vi "TDMS_LogMeasurements.vi"(8 "error in (no error)":errorcluster, 9 "Current Time":timestamp, 10 "Motor Measurements":T1, 11 "tdms file":refnum<k34>) -> (0 "error out":errorcluster, 3 "tdms file out":refnum<k34>)   [LabVIEW 2026]
uses:
  MotorMeasurements.ctl
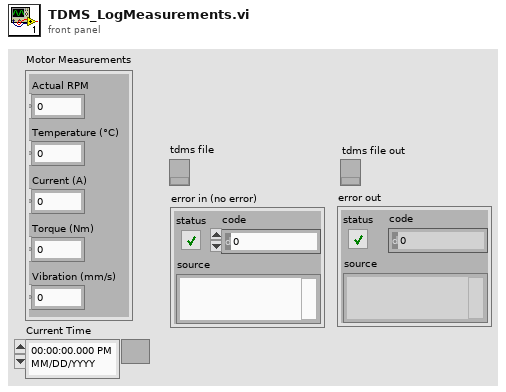
[diagram p1: front panel]
types:
  T1 = typedef "MotorMeasurements.ctl" = cluster{"Temperature (°C)":dbl, "Current (A)":dbl, "Torque (Nm)":dbl, "Vibration (mm/s)":dbl, "Actual RPM":dbl}
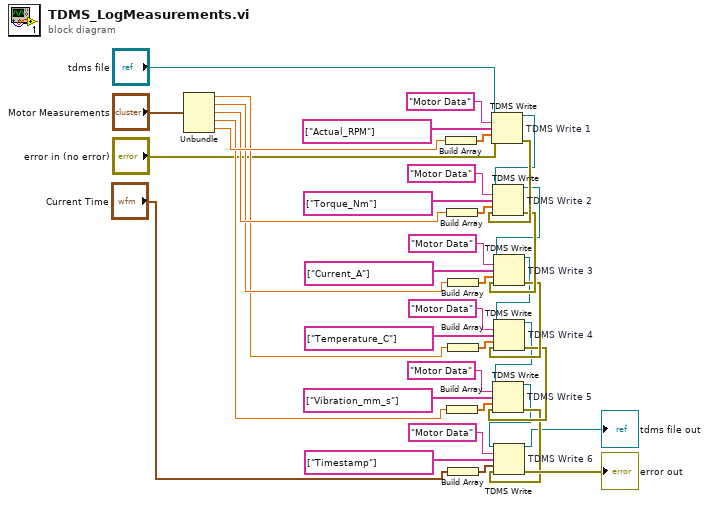
[diagram p0: block diagram]
diagram:
  n1 = Unbundle("Motor Measurements") -> ("Temperature (°C)"=w17:dbl, "Current (A)"=w18:dbl, "Torque (Nm)"=w19:dbl, "Vibration (mm/s)"=w9:dbl, "Actual RPM"=w20:dbl)
  n2 = Build Array(w20) -> (w35:dbl[])
  n3 = Build Array(w19) -> (w33:dbl[])
  n4 = Build Array(w9) -> (w22:dbl[])
  n5 = Build Array(w18) -> (w31:dbl[])
  n6 = Build Array(w17) -> (w37:dbl[])
  n7 = Build Array("Current Time") -> (w14:timestamp[])
  n8 = TDMS Write "TDMS Write 1"(0:"tdms file", 5:"Motor Data" ("group name in (Untitled)"), 7:string[] ["Actual_RPM"] ("channel name(s) in (Untitled)"), 9:w35, 11:"error in (no error)") -> (4:w6:refnum<k34>, 15:w27:errorcluster)  [unwired: 1 in, 2 out]
  n9 = TDMS Write "TDMS Write 2"(0:w6, 5:"Motor Data" ("group name in (Untitled)"), 7:string[] ["Torque_Nm"] ("channel name(s) in (Untitled)"), 9:w33, 11:w27) -> (4:w5:refnum<k34>, 15:w26:errorcluster)  [unwired: 1 in, 2 out]
  n10 = TDMS Write "TDMS Write 3"(0:w5, 5:"Motor Data" ("group name in (Untitled)"), 7:string[] ["Current_A"] ("channel name(s) in (Untitled)"), 9:w31, 11:w26) -> (4:w4:refnum<k34>, 15:w25:errorcluster)  [unwired: 1 in, 2 out]
  n11 = TDMS Write "TDMS Write 4"(0:w4, 5:"Motor Data" ("group name in (Untitled)"), 7:string[] ["Temperature_C"] ("channel name(s) in (Untitled)"), 9:w37, 11:w25) -> (4:w3:refnum<k34>, 15:w21:errorcluster)  [unwired: 1 in, 2 out]
  n12 = TDMS Write "TDMS Write 5"(0:w3, 5:"Motor Data" ("group name in (Untitled)"), 7:string[] ["Vibration_mm_s"] ("channel name(s) in (Untitled)"), 9:w22, 11:w21) -> (4:w2:refnum<k34>, 15:w12:errorcluster)  [unwired: 1 in, 2 out]
  n13 = TDMS Write "TDMS Write 6"(0:w2, 5:"Motor Data" ("group name in (Untitled)"), 7:string[] ["Timestamp"] ("channel name(s) in (Untitled)"), 9:w14, 11:w12) -> (4:→"tdms file out":refnum<k34>, 15:→"error out":errorcluster)  [unwired: 1 in, 2 out]
